vi "SwissSPAD Live_DAQ Parameters to Gate Configuration.vi"(9 "SS2 DAQ Parameters":T1 {"Sync Period" min=0.0 max=4.294967295; "# Sets" min=1}, 10 "Gate Configuration Name":string) -> (1 "Gate Configuration Definition out":T3)   [LabVIEW 2021]
uses:
  SwissSPAD Live_SS2 Gate Configuration.ctl
  SwissSPAD Live_SS2 Gate Definition.ctl
  SwissSPAD Live_SS2 DAQ Parameters 3.ctl
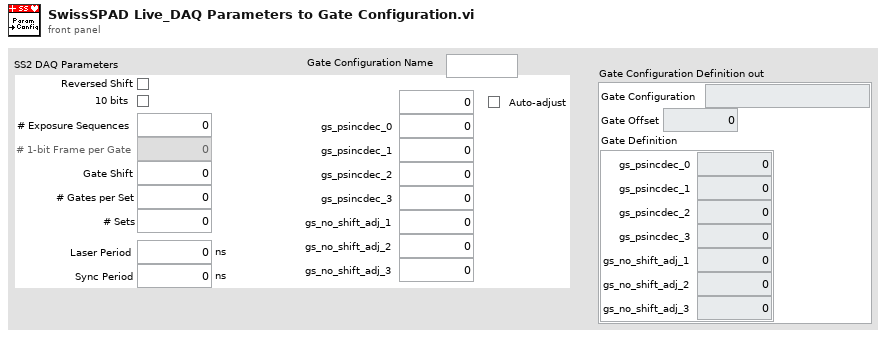
[diagram p1: front panel]
types:
  T1 = typedef "SwissSPAD Live_SS2 DAQ Parameters 3.ctl" = cluster{"10 bits":bool, "# Exposure Sequences":u32, "# 1-bit Frame per Gate":u32, "Gate Shift":u32, "# Gates per Set":u32, "# Sets":u32, "Laser Period":dbl[unit], "Sync Period":dbl[unit], "Gate Offset":u32, "Auto-adjust Gate Offset":bool, "Gate Definition":T2, "Reversed Shift":bool}
  T2 = typedef "SwissSPAD Live_SS2 Gate Definition.ctl" = cluster{"gs_psincdec_0":u32, "gs_psincdec_1":u32, "gs_psincdec_2":u32, "gs_psincdec_3":u32, "gs_no_shift_adj_1":u32, "gs_no_shift_adj_2":u32, "gs_no_shift_adj_3":u32}
  T3 = typedef "SwissSPAD Live_SS2 Gate Configuration.ctl" = cluster{"Gate Configuration":string, "Gate Offset":u32, "Gate Definition":T2}
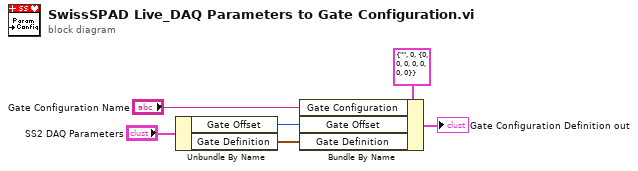
[diagram p0: block diagram]
diagram:
  n1 = Unbundle By Name("SS2 DAQ Parameters") -> ("Gate Offset"=w4:u32, "Gate Definition"=w5:T2)
  n2 = Bundle By Name(cluster=T3 {"Gate Configuration"="", "Gate Offset"=0, "Gate Definition"={"gs_psincdec_0"=0, "gs_psincdec_1"=0, "gs_psincdec_2"=0, "gs_psincdec_3"=0, "gs_no_shift_adj_1"=0, "gs_no_shift_adj_2"=0, "gs_no_shift_adj_3"=0}} ("Gate Configuration Definition in"), "Gate Configuration"="Gate Configuration Name", "Gate Offset"=w4, "Gate Definition"=w5) -> (→"Gate Configuration Definition out":T3)
